vi "Read Statement_id.vi"(11 "Result in":refnum<class "Result.lvclass">) -> (2 "Statement_id":i32, 3 "Result out":refnum<class "Result.lvclass">)   [LabVIEW 2018, in "InfluxDB Client.lvlib" / "Result.lvclass"]
uses:
  Result.lvclass
  Result.lvclass/Result.ctl
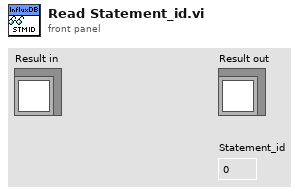
[diagram p1: front panel]
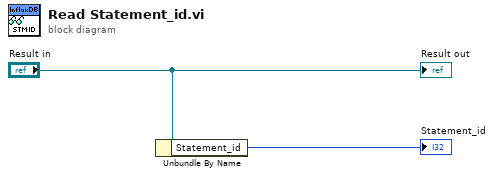
[diagram p0: block diagram]
diagram:
  n1 = Unbundle By Name("Result in") -> ("Statement_id"=→"Statement_id":i32)
  "Result out" <- "Result in"
